vi "Password.vi"(3 "ActivatePASSWView":bool) -> (0 "This VI":refnum<vi>, 1 "enable":bool)   [LabVIEW 2019, in "Logik.lvlib"]
uses:
  Logik.lvlib
panel:
  out "timer":u32
  in  "password":string
  in  "OK Button":bool
  # "Enter password:"
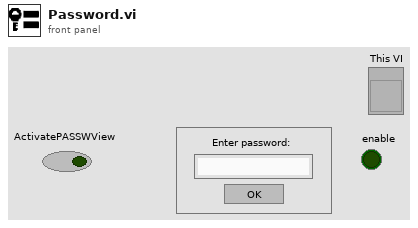
[diagram p1: front panel]
types:
  T1 = enum32{"Invalid", "Standard", "Closed", "Hidden", "Minimized", "Maximized"}
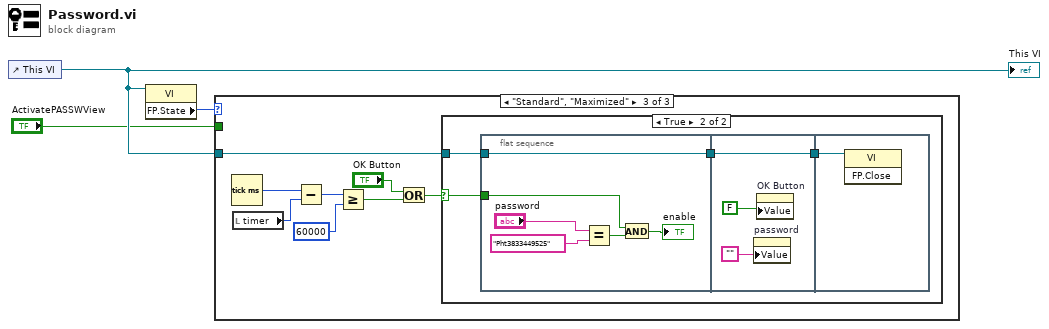
[diagram p0: block diagram]
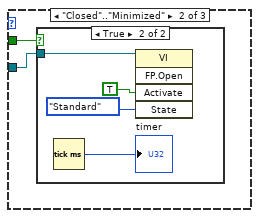
[diagram p3: hidden frame]
diagram:
  n1 = control-ref of="This VI"() -> (w2:refnum<vi>)
  "This VI" <- w2
  n2 = property class="VI"(reference=w2) -> ("FP.State"=w3:T1)  [unwired: 1 in, 2 out]
  n3 = case shown="\"Standard\", \"Maximized\"" w3 {
    tunnel: "ActivatePASSWView" -> [_ w5 _]
    tunnel: w2 -> [_ w4 w16]
    frame "Invalid", Default {
    }
    frame "Closed".."Minimized" {
      n4 = case shown="True" w5 {
        tunnel: w4 -> [_ w7]
        frame False {
        }
        frame True {
          n5 = Tick Count (ms)() -> (millisecond timer value=→"timer":u32)
          n6 = invoke class="VI" method="FP.Open"(reference=w7, "Activate"=TRUE ("Activate?"), "State"=T1."Standard") -> ()  [unwired: 2 in, 5 out]
        }
      }
    }
    frame "Standard", "Maximized" {
      n7 = Tick Count (ms)() -> (millisecond timer value=w12:u32)
      n8 = local read "timer"() -> (w11:u32)
      n9 = Subtract(x=w12, y=w11) -> (x-y=w10:u32)
      n10 = Greater Or Equal?(x=w10, y=u32 60000) -> (x >= y?=w13:bool)
      n11 = Or(x="OK Button", y=w13) -> (x .or. y?=w17:bool)
      n12 = case shown="True" w17 {
        selector: w17 -> [_ w21]
        tunnel: w16 -> [_ w18]
        frame False {
        }
        frame True {
          n13 = flat-sequence {
            tunnel: w21 -> [w24]
            tunnel: [w22] -> w19
            tunnel: w18 -> [w22]
            tunnel: [w28] -> w20
            tunnel: w19 -> [w28]
            tunnel: w20 -> [w31]
            frame #0 {
              n14 = Equal?(x="password", y="Pht3833449525" ("Edit Password 2")) -> (x = y?=w27:bool)
              n15 = And(x=w24, y=w27) -> (x .and. y?=→"enable":bool)
            }
            frame #1 {
              n16 = property on="password" class="Str"("Value"="") -> ()  [unwired: 2 in, 2 out]
              n17 = property on="OK Button" class="Bool"("Value"=FALSE) -> ()  [unwired: 2 in, 2 out]
            }
            frame #2 {
              n18 = invoke class="VI" method="FP.Close"(reference=w31) -> ()  [unwired: 2 in, 3 out]
            }
          }
        }
      }
    }
  }
